vi "Find Entity by ID.vi"(7 "Entity Type":refnum<class "Entity.lvclass">, 8 "error in (no error)":errorcluster, 10 "Entity ID":T1, 11 "Entity Manager in":refnum<class "Entity Manager.lvclass">) -> (0 "error out":errorcluster, 2 "Entity":refnum<class "Entity.lvclass">, 3 "Entity Manager out":refnum<class "Entity Manager.lvclass">)   [LabVIEW 2020, in "Conditum.lvlib" / "Entity Manager.lvclass"]
uses:
  Entity Manager.lvclass
  Database Platform/Database Platform.lvclass
  Entity/Entity.lvclass
  Entity ID.ctl
  Conditum.lvlib
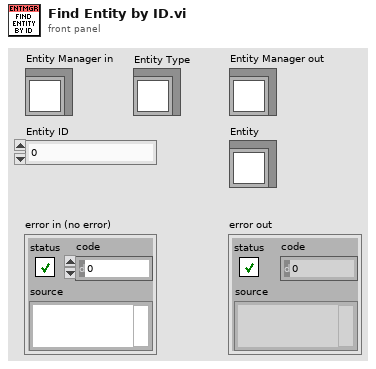
[diagram p1: front panel]
types:
  T1 = typedef "Conditum.lvlib/Entity ID.ctl" = i64
  T2 = typedef "Conditum.lvlib/Entity Manager.lvclass/Known Entity.ctl" = cluster{"Entity":refnum<class "Entity.lvclass">, "Types":refnum<class "Type.lvclass">[], "Type Name Map":map{string, i32}}
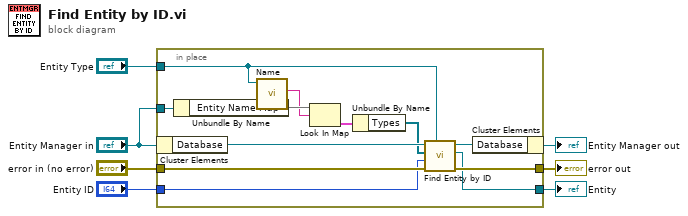
[diagram p0: block diagram]
diagram:
  n1 = in-place {
    in-place-border: "Entity ID" -> [w10]
    in-place-border: "error in (no error)" -> [w17]
    in-place-border: "Entity Type" -> [w14]
    in-place-border: [w16] -> w4
    in-place-border: [w15] -> w2
    in-place-border: "Entity Manager in" -> [w8]
    n2 = in-place-cluster #1("Entity Manager in") -> ("Database"=w19:refnum<class "Database Platform.lvclass">)
    n3 = Unbundle By Name(w8) -> ("Entity Name Map"=w13:map{string, T2})
    n4 = call-dynamic "Name.vi"("Entity in"=w14) -> ("Name"=w12:string)  [unwired: 10 in]
    n5 = Look In Map(map=w13, key=w12) -> (value=w11:T2)  [unwired: 1 in, 1 out]
    n6 = Unbundle By Name(w11) -> ("Types"=w9:refnum<class "Type.lvclass">[])
    n7 = call "Find Entity by ID.vi"("Entity Type"=w14, "error in (no error)"=w17, "Entity ID"=w10, "Types"=w9, "Database in"=w19) -> ("error out"=w16:errorcluster, "Entity"=w15:refnum<class "Entity.lvclass">, "Database out"=w18:refnum<class "Database Platform.lvclass">)  [unwired: 4 in]
    n8 = in-place-cluster #1("Database"=w18) -> (→"Entity Manager out":refnum<class "Entity Manager.lvclass">)
  }
  "error out" <- w4
  "Entity" <- w2
